vi "Current System Status.vi"(8 "error in":errorcluster, 11 "IP address":string) -> (0 "error out":errorcluster, 1 "Requires Update?":string, 2 "ImageTitle":string, 3 "Firmware Version":string)   [LabVIEW 2020]
uses:
  <vilib>/nisyscfg/Get Installed Set.vi
  <vilib>/nisyscfg/Close (System).vi
  <resource>/objmgr/nisysapi.rc
  <vilib>/nisyscfg/nisyscfg.lvlib
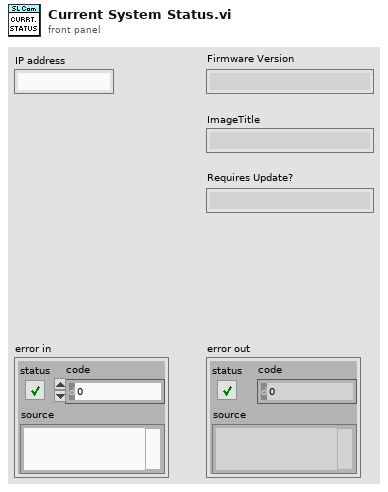
[diagram p1: front panel]
types:
  T1 = typedef "nisyscfg.lvlib/Software Set 1.2.ctl" = cluster{"information":T2, "items":T2[], "add-ons":T2[]}
  T2 = typedef "nisyscfg.lvlib/Software 1.2.ctl" = cluster{"title":string, "description":string, "ID":string, "version":string, "component type":T3}
  T3 = typedef "nisyscfg.lvlib/Component Type.ctl" = u32
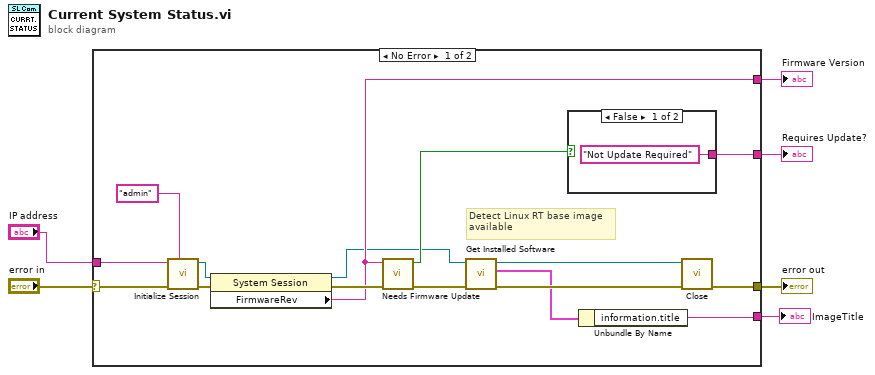
[diagram p0: block diagram]
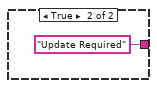
[diagram p2: hidden frame]
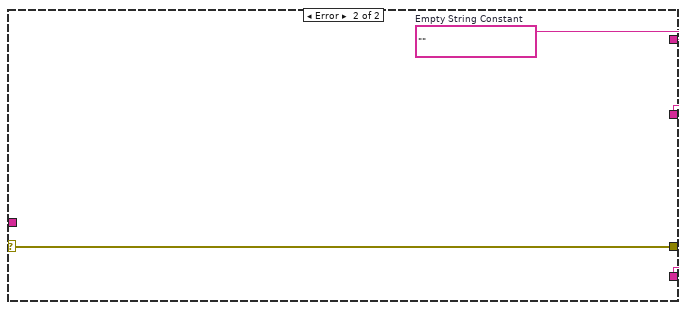
[diagram p3: hidden frame]
diagram:
  n1 = case shown="No Error" "error in" {
    selector: "error in" -> [w13 w26]
    tunnel: [w22 w26] -> w6
    tunnel: "IP address" -> [w21 _]
    tunnel: [w15 w25] -> w4
    tunnel: [w14 w25] -> w3
    tunnel: [w7 w25] -> w1
    frame No Error {
      # "Detect Linux RT base image\navailable"
      n2 = call <vilib>:"Initialize Session.vi"("User Name"="admin", "error in (no error)"=w13, "Target (localhost)"=w21) -> ("error out"=w19:errorcluster, "Session out"=w18:refnum<k21>)  [unwired: 7 in]
      n3 = property class="System Session"(reference=w18, error in=w19) -> (reference out=w12:refnum<k21>, error out=w17:errorcluster, "FirmwareRev"=w14:string)
      n4 = call "Needs Firmware Update.vi"("error in (no error)"=w17, "FirmwareRev"=w14) -> ("error out"=w9:errorcluster, "Update?"=w16:bool)  [unwired: 8 in]
      n5 = call-poly <vilib>:"Get Installed Software.vi"("error in (no error)"=w9, "Session in"=w12) -> ("error out"=w10:errorcluster, "Software Set"=w8:T1, "Session out"=w11:refnum<k21>)  [unwired: 7 in]
      n6 = case shown="False" w16 {
        tunnel: ["Not Update Required" ("Requires Update?") "Update Required" ("Requires Update?")] -> w15
        frame False {
        }
        frame True {
        }
      }
      n7 = Unbundle By Name(w8) -> ("information.title"=w7:string)
      n8 = call-poly <vilib>:"Close.vi"("error in (no error)"=w10, "Session in"=w11) -> ("error out"=w22:errorcluster)  [unwired: 9 in]
    }
    frame Error {
      w25 = ""  # Empty String Constant
    }
  }
  "error out" <- w6
  "Firmware Version" <- w3
  "Requires Update?" <- w4
  "ImageTitle" <- w1
